vi "Find Nearest Point.vi"(10 "xy point (units)":cluster{"x":dbl, "y":dbl}, 11 "cartesian data":T1) -> (1 "col":i32, 2 "row":i32, 3 "distance":dbl)   [LabVIEW 2017, in "NI_Robotics_2D Rangefinder Picture.lvlib"]
uses:
  <vilib>/robotics/Controls/2D Rangefinder/2D Rangefinder Picture/NI_Robotics_2D Rangefinder Picture.lvlib
  <vilib>/robotics/Controls/2D Rangefinder/2D Rangefinder Picture/Cartesian Data.ctl
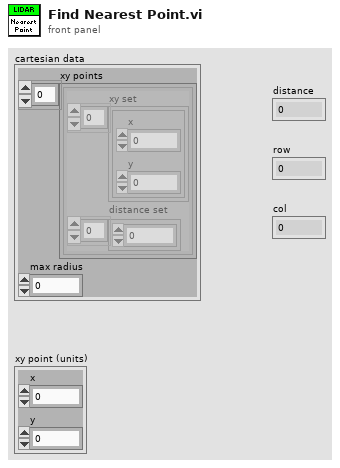
[diagram p1: front panel]
types:
  T1 = typedef "NI_Robotics_2D Rangefinder Picture.lvlib/Cartesian Data.ctl" = cluster{"xy points":cluster{"xy set":cluster{"x":dbl, "y":dbl}[], "distance set":dbl[]}[], "max radius":dbl}
  T2 = cluster{"xy set":cluster{"x":dbl, "y":dbl}[], "distance set":dbl[]}[]
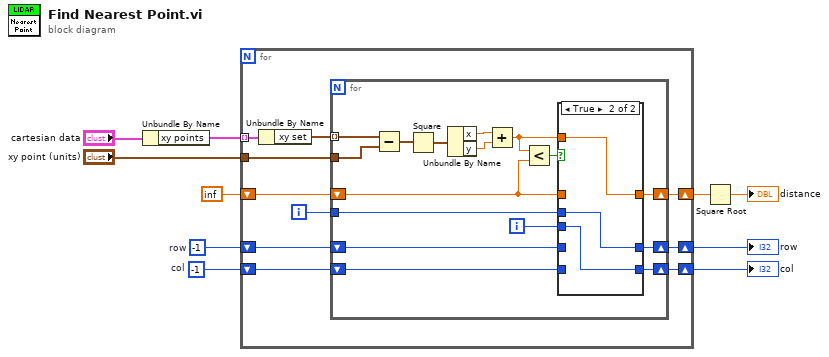
[diagram p0: block diagram]
diagram:
  w5 = -1  # col
  w6 = -1  # row
  n1 = Unbundle By Name("cartesian data") -> ("xy points"=w9:T2)
  n2 = for {
    tunnel: w9 -> [w20] mode=indexing
    tunnel: "xy point (units)" -> [w18]
    shift-right: [w15] -> w2
    shift-left: inf -> [w17]
    shift-right: [w12] -> w4
    shift-left: w6 -> [w14]
    shift-right: [w11] -> w3
    shift-left: w5 -> [w13]
    i -> [w16]
    n3 = Unbundle By Name(w20) -> ("xy set"=w19:cluster{"x":dbl, "y":dbl}[])
    n4 = for {
      tunnel: w19 -> [w36] mode=indexing
      tunnel: w18 -> [w35]
      shift-right: [w28] -> w15
      shift-left: w17 -> [w29]
      tunnel: w16 -> [w21]
      shift-right: [w26] -> w12
      shift-left: w14 -> [w27]
      shift-right: [w24] -> w11
      shift-left: w13 -> [w25]
      i -> [w23]
      n5 = Subtract(x=w36, y=w35) -> (x-y=w34:cluster{"x":dbl, "y":dbl})
      n6 = Square(x=w34) -> (x^2=w33:cluster{"x":dbl, "y":dbl})
      n7 = Unbundle By Name(w33) -> ("x"=w32:dbl, "y"=w31:dbl)
      n8 = Add(x=w32, y=w31) -> (x+y=w22:dbl)
      n9 = Less?(x=w22, y=w29) -> (x < y?=w30:bool)
      n10 = case shown="True" w30 {
        tunnel: w29 -> [w39 _]
        tunnel: [w39 w42] -> w28
        tunnel: w27 -> [w38 _]
        tunnel: [w38 w41] -> w26
        tunnel: w25 -> [w37 _]
        tunnel: [w37 w40] -> w24
        tunnel: w23 -> [_ w40]
        tunnel: w22 -> [_ w42]
        tunnel: w21 -> [_ w41]
        frame False {
        }
        frame True {
        }
      }
    }
  }
  "row" <- w4
  "col" <- w3
  n11 = Square Root(x=w2) -> (sqrt(x)=→"distance":dbl)
